vi "PreCloseDevice.vi"(10 "Send Thread":refnum<vi>, 11 "Update Thread":refnum<vi>) -> ()   [LabVIEW 2011]
panel:
  # "先关闭校验线程、发送线程、接收线程。"
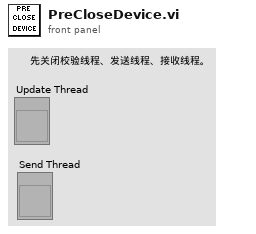
[diagram p1: front panel]
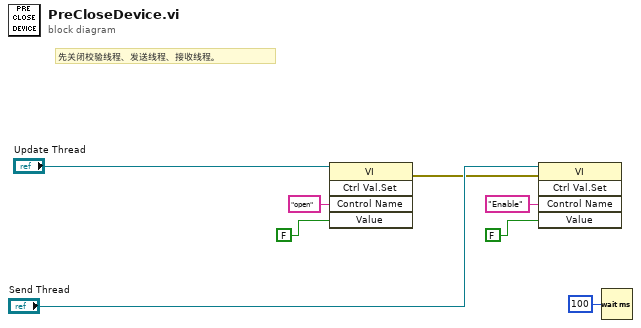
[diagram p0: block diagram]
diagram:
  # "先关闭校验线程、发送线程、接收线程。"
  n1 = invoke class="VI" method="Ctrl Val.Set"(reference="Update Thread", "Control Name"="open" ("控件名"), "Value"=FALSE) -> (error out=w2:errorcluster)  [unwired: 2 in, 4 out]
  n2 = invoke class="VI" method="Ctrl Val.Set"(reference="Send Thread", error in=w2, "Control Name"="Enable" ("控件名"), "Value"=FALSE) -> ()  [unwired: 1 in, 5 out]
  n3 = Wait (ms)(milliseconds to wait=u32 100 ("等待时间（毫秒）")) -> ()  [unwired: 1 out]
